vi "initialize eip tag lists.vi"(4 "output dictionary":refnum<class "data dictionary.lvclass">, 6 "input dictionary":refnum<class "data dictionary.lvclass">, 8 "error in":errorcluster, 10 "EthernetIP configuration in":refnum<class "EIP Tags Configuration.lvclass">, 11 "EthernetIP runtime in":refnum<class "EIP Tags Runtime.lvclass">) -> (0 "error out":errorcluster, 3 "EthernetIP runtime out":refnum<class "EIP Tags Runtime.lvclass">)   [LabVIEW 2013, in "EIP Tags Runtime.lvclass"]
uses:
  EIP Tags Runtime.lvclass
  configuration/EIP Tags Configuration.lvclass
  <vilib>/NI/Tag Bus/dictionary/data dictionary.lvclass
  <vilib>/ethernetip/ethernetip.llb/ethernetip.ctl
  configuration/EIP Tags Configuration.lvclass/EIP Tags Configuration.ctl
  eip tag spec.ctl
  configuration/eip tag types.ctl
  channel/EIP Tags Channel.lvclass/EIP Tags Channel.ctl
  <vilib>/NI/Tag Bus Module Framework/channel/TBM channel.lvclass/TBM channel.ctl
  <vilib>/NI/Tag Bus/tag/tag descriptor.lvclass/tag descriptor.ctl
  EIP Tags Runtime.lvclass/EIP Tags Runtime.ctl
  channel/Read EIP Tag UUID.vi
  <vilib>/NI/Tag Bus Module Framework/channel/Read channel classification.vi
  <vilib>/NI/Tag Bus/tag/read tag name.vi
  <vilib>/NI/Tag Bus/tag/read data type.vi
  channel/Read element.vi
  configuration/Read Timeout (ms).vi
  configuration/Read EIP tags.vi
  configuration/read eip channels.vi
  <vilib>/ethernetip/ethernetip.llb/EthernetIP Tag Read Raw.vi
  channel/EIP Tags Channel.lvclass
  <vilib>/ethernetip/ethernetip.lvlib
  <vilib>/NI/Configuration Framework/NISE_CEF_TreeControl.lvlib
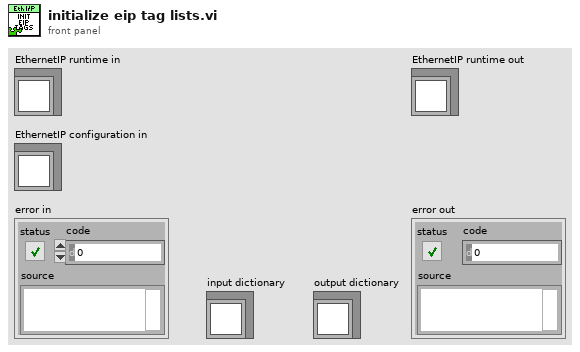
[diagram p1: front panel]
types:
  T1 = typedef "ethernetip.lvlib/ethernetip.ctl" = refnum<k21>
  T2 = typedef "EIP Tags Configuration.lvclass/eip tag definition.ctl" = cluster{"eip tag types":T3, "unique tag name":string, "Number of Elements":u32}
  T3 = typedef "EIP Tags Configuration.lvclass/eip tag types.ctl" = enum16{"SINT", "INT", "DINT", "REAL", "BOOL", "STRING"}
  T4 = typedef "EIP Tags Runtime.lvclass/eip tag spec.ctl" = cluster{"eip tag types":T3, "Network Path":string, "Tag Name":string, "Number of Elements":u32, "data indices":i32[], "tag bus indices":i32[]}
  T5 = typedef "TBM channel.lvclass/channel classification.ctl" = enum16{"input data", "output data", "processing parameter", "processing result"}
  T6 = typedef "tag bus.lvlib/tag descriptor.lvclass/Data Type.ctl" = enum16{"Double", "Single", "I64", "I32", "I16", "I8", "U64", "U32", "U16", "U8", "Boolean", "String", "Array of Double", "Array of Single", "Array of I64", "Array of I32", "Array of I16", "Array of I8", "Array of U64", "Array of U32", "Array of U16", "Array of U8", "Array of Boolean", "Array of String"}
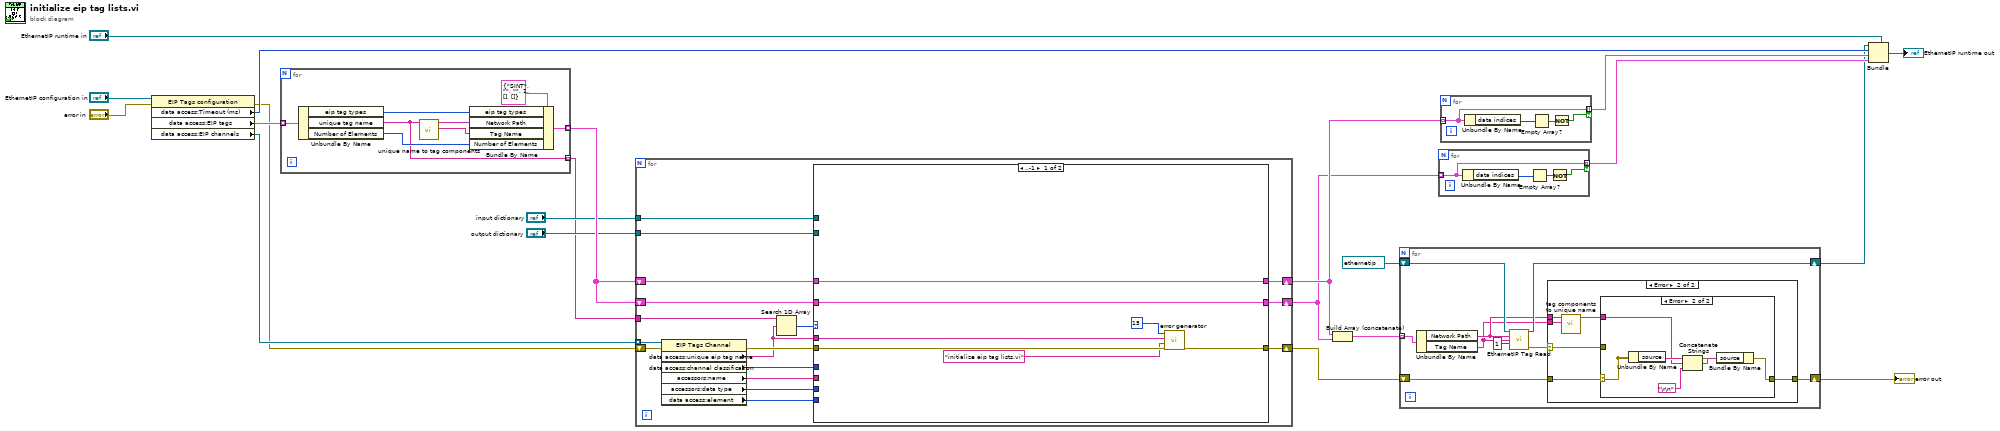
[diagram p0: block diagram]
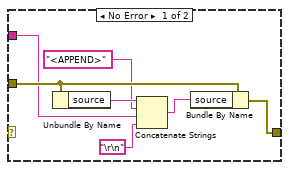
[diagram p3: hidden frame]
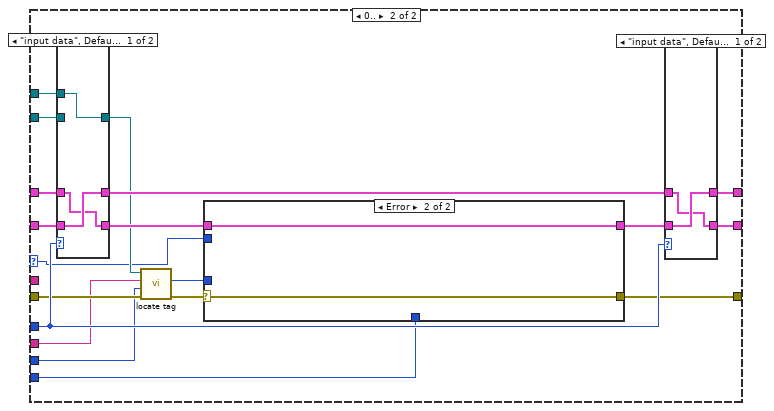
[diagram p4: hidden frame]
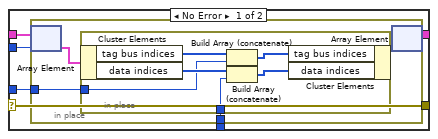
[diagram p5: hidden frame]
diagram:
  n1 = property class="EIP Tags configuration"(reference="EthernetIP configuration in", error in="error in") -> (error out=w11:errorcluster, "data access:Timeout (ms)"=w17:i32, "data access:EIP tags"=w16:T2[], "data access:EIP channels"=w14:refnum<class "EIP Tags Channel.lvclass">[])  [unwired: 1 out]
  n2 = for {
    tunnel: w16 -> [w29] mode=indexing
    tunnel: [w23] -> w15 mode=indexing
    tunnel: [w22] -> w8 mode=indexing
    n3 = Unbundle By Name(w29) -> ("eip tag types"=w27:T3, "unique tag name"=w22:string, "Number of Elements"=w26:u32)
    n4 = call "unique name to tag components.vi"("unique name"=w22) -> ("Tag Name"=w24:string, "Network Path"=w25:string)  [unwired: 9 in]
    n5 = Bundle By Name(cluster=T4 {"eip tag types"=enum."SINT", "Network Path"="", "Tag Name"="", "Number of Elements"=1, "data indices"=[], "tag bus indices"=[]} ("tag spec"), "eip tag types"=w27, "Network Path"=w25, "Tag Name"=w24, "Number of Elements"=w26) -> (w23:T4)
  }
  n6 = for {
    shift-right: [w41] -> w5
    shift-left: w15 -> [w42]
    shift-right: [w39] -> w4
    shift-left: w15 -> [w40]
    tunnel: w14 -> [w45] mode=indexing
    tunnel: "input dictionary" -> [w36]
    tunnel: "output dictionary" -> [w35]
    shift-right: [w37] -> w2
    shift-left: w11 -> [w46]
    tunnel: w8 -> [w44]
    n7 = property class="EIP Tags Channel"(reference=w45, error in=w46) -> (error out=w38:errorcluster, "data access:unique eip tag name"=w34:string, "data access:channel classification"=w33:T5, "accessors:name"=w31:string, "accessors:data type"=w30:T6, "data access:element"=w32:i32)  [unwired: 1 out]
    n8 = Search 1D Array(1D array=w44, element=w34) -> (index of element=w43:i32)  [unwired: 1 in]
    n9 = case shown="..-1" w43 {
      selector: w43 -> [_ w56]
      tunnel: w42 -> [w53 w70]
      tunnel: [w53 w68] -> w41
      tunnel: w40 -> [w52 w69]
      tunnel: [w52 w67] -> w39
      tunnel: w38 -> [w51 w62]
      tunnel: [w50 w57] -> w37
      tunnel: w36 -> [_ w71]
      tunnel: w35 -> [_ w72]
      tunnel: w34 -> [w48 _]
      tunnel: w33 -> [_ w65]
      tunnel: w32 -> [_ w54]
      tunnel: w31 -> [_ w60]
      tunnel: w30 -> [_ w59]
      frame ..-1 {
        n10 = call <vilib>:"error generator.vi"("error in"=w51, "source"="initialize eip tag lists.vi", "append error message"=w48, "error code (0)"=15) -> ("error out"=w50:errorcluster)  [unwired: 5 in]
      }
      frame 0.. {
        n11 = case shown="\"input data\", Default" w65 {
          tunnel: [w97 w100] -> w61
          tunnel: w72 -> [_ w100]
          tunnel: w71 -> [w97 _]
          tunnel: w70 -> [w95 w98]
          tunnel: w69 -> [w96 w99]
          tunnel: [w95 w99] -> w64
          tunnel: [w96 w98] -> w66
          frame "input data", Default {
          }
          frame "output data" {
          }
        }
        n12 = call <vilib>:"locate tag.vi"("error in"=w62, "data type"=w59, "name"=w60, "data dictionary in"=w61) -> ("error out"=w58:errorcluster, "index"=w55:i32)  [unwired: 5 in, 1 out]
        n13 = case shown="Error" w58 {
          selector: w58 -> [w76 w90]
          tunnel: w64 -> [w78 w89]
          tunnel: [w77 w89] -> w63
          tunnel: [w76 w90] -> w57
          tunnel: w56 -> [w75 _]
          tunnel: w55 -> [w74 _]
          tunnel: w54 -> [w73 _]
          frame No Error {
            n14 = in-place {
              in-place-border: w74 -> [w80]
              in-place-border: w73 -> [w79]
              n15 = in-place-array #1(w78, w75) -> (w82:T4)
              n16 = in-place {
                in-place-border: w80 -> [w84]
                in-place-border: w79 -> [w83]
                n17 = in-place-cluster #2(w82) -> ("tag bus indices"=w87:i32[], "data indices"=w88:i32[])
                n18 = Build Array (concatenate)(w87, w84) -> (w86:i32[])
                n19 = Build Array (concatenate)(w88, w83) -> (w85:i32[])
                n20 = in-place-cluster #2("tag bus indices"=w86, "data indices"=w85) -> (w81:T4)
              }
              n21 = in-place-array #1(w81) -> (w77:T4[])  [unwired: 1 out]
            }
          }
          frame Error {
          }
        }
        n22 = case shown="\"input data\", Default" w65 {
          tunnel: w66 -> [w91 w93]
          tunnel: w63 -> [w92 w94]
          tunnel: [w91 w94] -> w67
          tunnel: [w92 w93] -> w68
          frame "input data", Default {
          }
          frame "output data" {
          }
        }
      }
    }
  }
  n23 = Build Array (concatenate)(w5, w4) -> (w3:T4[])
  n24 = for {
    shift-right: [w108] -> w6
    shift-left: T1 "Default" ("Session in") -> [w109]
    tunnel: w3 -> [w107] mode=indexing
    shift-right: [w104] -> w1
    shift-left: w2 -> [w103]
    n25 = Unbundle By Name(w107) -> ("Network Path"=w102:string, "Tag Name"=w101:string)
    n26 = call-poly <vilib>:"EthernetIP Tag Read.vi"("Session in"=w109, "Network Path"=w102, "Tag Name"=w101, "Number of Elements"=u32 1) -> ("Session out"=w108:T1, "error out"=w105:errorcluster)  [unwired: 9 in, 1 out]
    n27 = case shown="Error" w105 {
      selector: w105 -> [_ w114]
      tunnel: [w110 w115] -> w104
      tunnel: w103 -> [w110 w116]
      tunnel: w102 -> [_ w113]
      tunnel: w101 -> [_ w112]
      frame No Error {
      }
      frame Error {
        n28 = call "tag components to unique name.vi"("Tag Name"=w112, "Network Path"=w113) -> ("unique name"=w111:string)  [unwired: 9 in]
        n29 = case shown="Error" w116 {
          selector: w116 -> [_ w124]
          tunnel: [w122 w129] -> w115
          tunnel: w114 -> [w123 _]
          tunnel: w111 -> [w117 w125]
          frame No Error {
            n30 = Unbundle By Name(w123) -> ("source"=w120:string)
            n31 = Concatenate Strings(w120, "<APPEND>" ("string"), w117, "\r\n") -> (w121:string)
            n32 = Bundle By Name(cluster=w123, "source"=w121) -> (w122:errorcluster)
          }
          frame Error {
            n33 = Unbundle By Name(w124) -> ("source"=w127:string)
            n34 = Concatenate Strings(w127, w125, "\r\n") -> (w128:string)
            n35 = Bundle By Name(cluster=w124, "source"=w128) -> (w129:errorcluster)
          }
        }
      }
    }
  }
  "error out" <- w1
  n36 = for {
    tunnel: w4 -> [w131] mode=indexing
    tunnel: [w131] -> w9 mode=indexing if=w130
    n37 = Unbundle By Name(w131) -> ("data indices"=w133:i32[])
    n38 = Empty Array?(array=w133) -> (empty?=w132:bool)
    n39 = Not(x=w132) -> (.not. x?=w130:bool)
  }
  n40 = for {
    tunnel: w5 -> [w135] mode=indexing
    tunnel: [w135] -> w10 mode=indexing if=w134
    n41 = Unbundle By Name(w135) -> ("data indices"=w137:i32[])
    n42 = Empty Array?(array=w137) -> (empty?=w136:bool)
    n43 = Not(x=w136) -> (.not. x?=w134:bool)
  }
  n44 = Bundle(cluster="EthernetIP runtime in", w6, w17, w10, w9) -> (→"EthernetIP runtime out":refnum<class "EIP Tags Runtime.lvclass">)
